vi "SVFA Unit Conversion (1 Ch).vi"(0 "spectrum":cluster{"x0":dbl, "dx":dbl, "magnitude":dbl[]} {"magnitude" format="%.2p"; "dx" format="%.2p"; "x0" format="%.2p"}, 1 "desired scaling":T2 {"dB reference (0: no change)" format="%.2f"}, 2 "spectral density desired":T1(ring), 4 "spectrum info in":T3={"channel name"="", "description"="", "x-axis units"=0, "spectral info"={"spectrum type"=enum."Power [Magnitude^2]", "linear/dB"=enum."linear", "window"=0, "window size"=0, "FFT size"=0}, "engineering units"=0, "custom label"="", "dB reference [EU]"=0.0, "peak units"=enum."rms", "weighting filter"=0, "spectral density?"=FALSE, "unit label"="", "spectrum skewed?"=FALSE, "complimentary spectrum units"=enum."none"} {"x-axis units" items=["Time (s)"=0, "Frequency-CB (Hz)"=1, "Frequency-CPB (Hz)"=1248, "Frequency-Arbitrary (Hz)"=2357, "Quefrency (s)"=2, "Revolutions (rev)"=3, "Order"=4, "Speed (RPM)"=11, "Speed (rad/s)"=21, "Index"=65535]; "weighting filter" items=["Linear", "A-weighting", "B-weighting", "C-weighting", "ITU-R 468-4", "Dolby", "CCITT", "C-message", "Wb", "Wc", "Wd", "We", "Wf", "Wh", "Wj", "Wk", "Wm", "AES17 20 kHz lowpass", "AES17 40 kHz lowpass", "AES17 20 kHz highpass", "AES17 40 kHz highpass"]; "dB reference [EU]" format="%.2f"; "engineering units" items=["custom..."=0, "V"=1, "A"=21, "C"=30, "pC"=31, "s"=32, "-"=29, "Pa"=2, "N"=20, "g"=3, "m/s^2"=4, "m/s"=5, "m"=6, "mm/s"=12, "mm"=13, "micron/s"=14, "micron"=15, "in/s^2"=7, "in/s"=8, "in"=9, "mil/s"=10, "mil"=11, "rad/s^2"=16, "rad/s"=17, "rad"=18, "deg/s^2"=26, "deg/s"=27, "deg"=28, "RPM"=22, "cycle/s^2"=23, "Hz"=24, "cycle"=25, "strain"=19]; "spectral info"."window" items=["None "=0, "Hanning"=1, "Hamming"=2, "Blackman-Harris"=3, "Exact Blackman"=4, "Blackman"=5, "Flat Top"=6, "4 Term B-Harris "=7, "7 Term B-Harris"=8, "Low Sidelobe"=9, "Force - Exponential"=10, "Gaussian"=62]}, 5 "error in (no error)":errorcluster) -> (14 "converted spectrum":cluster{"x0":dbl, "dx":dbl, "magnitude":dbl[]} {"magnitude" format="%.2p"; "dx" format="%.2p"; "x0" format="%.2p"}, 15 "unit label":string, 18 "spectrum info out":T3={"channel name"="", "description"="", "x-axis units"=0, "spectral info"={"spectrum type"=enum."Power [Magnitude^2]", "linear/dB"=enum."linear", "window"=0, "window size"=0, "FFT size"=0}, "engineering units"=0, "custom label"="", "dB reference [EU]"=0.0, "peak units"=enum."rms", "weighting filter"=0, "spectral density?"=FALSE, "unit label"="", "spectrum skewed?"=FALSE, "complimentary spectrum units"=enum."none"} {"x-axis units" items=["Time (s)"=0, "Frequency-CB (Hz)"=1, "Frequency-CPB (Hz)"=1248, "Frequency-Arbitrary (Hz)"=2357, "Quefrency (s)"=2, "Revolutions (rev)"=3, "Order"=4, "Speed (RPM)"=11, "Speed (rad/s)"=21, "Index"=65535]; "weighting filter" items=["Linear", "A-weighting", "B-weighting", "C-weighting", "ITU-R 468-4", "Dolby", "CCITT", "C-message", "Wb", "Wc", "Wd", "We", "Wf", "Wh", "Wj", "Wk", "Wm", "AES17 20 kHz lowpass", "AES17 40 kHz lowpass", "AES17 20 kHz highpass", "AES17 40 kHz highpass"]; "dB reference [EU]" format="%.2f"; "engineering units" items=["custom..."=0, "V"=1, "A"=21, "C"=30, "pC"=31, "s"=32, "-"=29, "Pa"=2, "N"=20, "g"=3, "m/s^2"=4, "m/s"=5, "m"=6, "mm/s"=12, "mm"=13, "micron/s"=14, "micron"=15, "in/s^2"=7, "in/s"=8, "in"=9, "mil/s"=10, "mil"=11, "rad/s^2"=16, "rad/s"=17, "rad"=18, "deg/s^2"=26, "deg/s"=27, "deg"=28, "RPM"=22, "cycle/s^2"=23, "Hz"=24, "cycle"=25, "strain"=19]; "spectral info"."window" items=["None "=0, "Hanning"=1, "Hamming"=2, "Blackman-Harris"=3, "Exact Blackman"=4, "Blackman"=5, "Flat Top"=6, "4 Term B-Harris "=7, "7 Term B-Harris"=8, "Low Sidelobe"=9, "Force - Exponential"=10, "Gaussian"=62]}, 19 "error out":errorcluster)   [LabVIEW 2017]
doc: "Converts between dB/linear, magnitude/magnitude^2, rms/peak/peak-peak, spectrum/spectral density, and dB ref1/dB ref2. Wire data to the <B>spectrum</B> input to determine the polymorphic instance to use or manually select the instance."
uses:
  <vilib>/addons/_NISVFA/_Shared subVIs/Controls/svc_Spectrum Info.ctl
  <vilib>/addons/_NISVFA/_Shared subVIs/Controls/svc_X-Axis Units.ctl
  <vilib>/addons/_NISVFA/_Shared subVIs/Controls/svc_Spectrum Type.ctl
  <vilib>/addons/_NISVFA/_Shared subVIs/Controls/svc_Engineering Units Text Ring.ctl
  <vilib>/addons/_NISVFA/_Shared subVIs/Controls/svc_Weighting Filter Text Ring.ctl
  <vilib>/addons/_NISVFA/_Shared subVIs/Controls/svc_Complimentary Spectrum Units.ctl
  <vilib>/addons/_NISVFA/_Spectrum Processing/subVIs/svfa_Peak to RMS to Peak2Peak.vi
  <vilib>/addons/_NISVFA/_Spectrum Processing/subVIs/svfa_Mag to Mag2.vi
  <vilib>/addons/_NISVFA/_Spectrum Processing/subVIs/svfa_Linear to dB.vi
  <vilib>/addons/_NISVFA/_Spectrum Processing/subVIs/svfa_dBrefA to dBrefB.vi
  <vilib>/addons/_NISVFA/_Spectrum Processing/subVIs/svfa_Spectrum to Spectral Density.vi
  <vilib>/addons/_NISVFA/_Shared subVIs/Common/svc_Get Weighting Enum and Labels.vi
  <vilib>/addons/_NISVFA/_Shared subVIs/Common/svc_Unit Label Lexical Class.vi
  <vilib>/addons/_NISVFA/_Shared subVIs/Common/svc_Engineering Units to Unit Label.vi
  <vilib>/addons/_NISVFA/_Shared subVIs/Common/svc_Format Value (DBL).vi
  <vilib>/addons/_NISVFA/_Shared subVIs/Common/svc_Window Parameters.vi
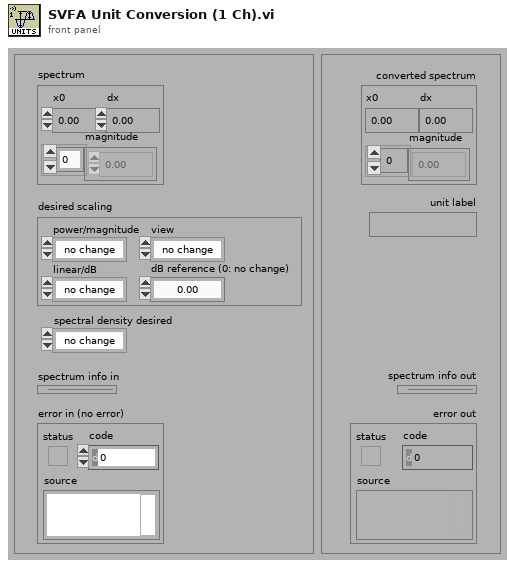
[diagram p1: front panel]
types:
  T1 = enum16{"no change", "spectrum", "spectral density"}
  T2 = cluster{"linear/dB":enum16{"no change", "linear", "dB"}, "dB reference (0: no change)":dbl, "power/magnitude":enum16{"no change", "power", "magnitude"}, "view":enum16{"no change", "rms", "peak", "peak-peak"}}
  T3 = typedef "svc_Spectrum Info.ctl" = cluster{"channel name":string, "description":string, "x-axis units":T4, "spectral info":cluster{"spectrum type":T5, "linear/dB":enum16{"linear", "dB"}, "window":u16, "window size":i32, "FFT size":i32}, "engineering units":T6, "custom label":string, "dB reference [EU]":dbl, "peak units":enum16{"rms", "peak", "peak-peak"}, "weighting filter":T7, "spectral density?":bool, "unit label":string, "spectrum skewed?":bool, "complimentary spectrum units":T8}
  T4 = typedef "svc_X-Axis Units.ctl" = u16
  T5 = typedef "svc_Spectrum Type.ctl" = enum16{"FFT Spectrum [complex]", "Amplitude [Magnitude]", "Power [Magnitude^2]", "Cross Spectrum [complex]", "Frequency Response [Complex]"}
  T6 = typedef "svc_Engineering Units Text Ring.ctl" = u16
  T7 = typedef "svc_Weighting Filter Text Ring.ctl" = u16
  T8 = typedef "svc_Complimentary Spectrum Units.ctl" = enum16{"none", "radians", "degrees", "cycles", "imaginary"}
  T9 = cluster{"linear/dB":bool, "dB reference (0: no change)":bool, "power/magnitude":bool, "view":bool}
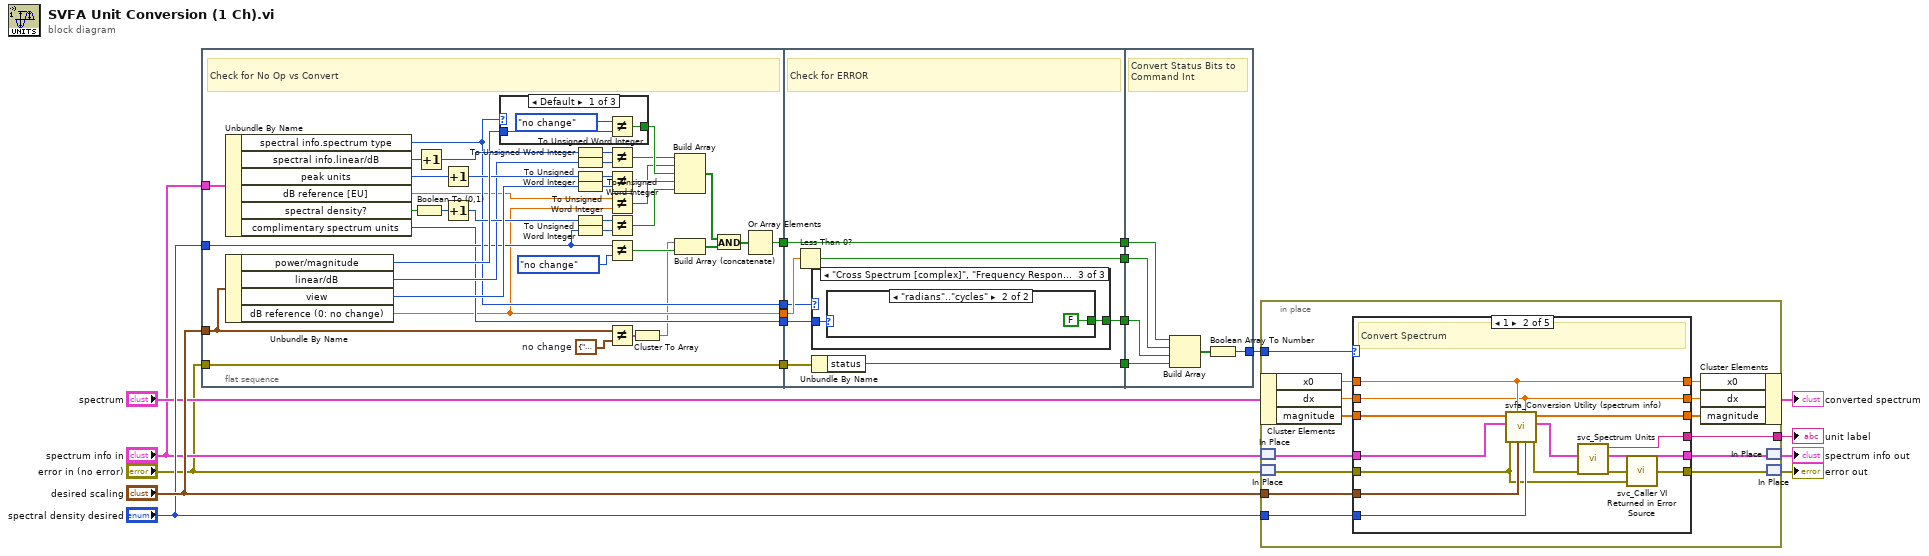
[diagram p0: block diagram]
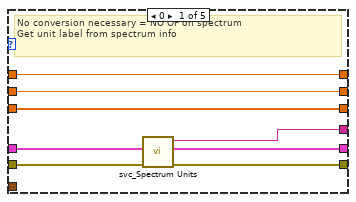
[diagram p2: hidden frame]
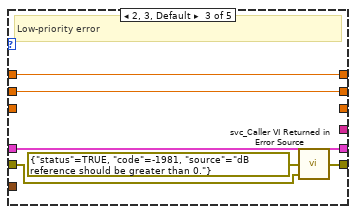
[diagram p3: hidden frame]
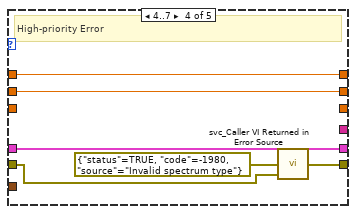
[diagram p4: hidden frame]
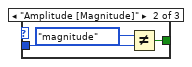
[diagram p6: hidden frame]
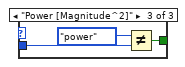
[diagram p7: hidden frame]
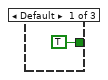
[diagram p8: hidden frame]
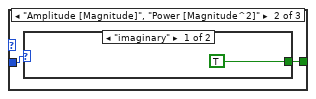
[diagram p9: hidden frame]
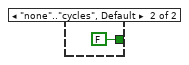
[diagram p10: hidden frame]
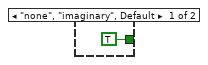
[diagram p11: hidden frame]
diagram:
  n1 = flat-sequence "Check for No Op vs Convert" {
    tunnel: "desired scaling" -> [w39]
    tunnel: "spectrum info in" -> [w57]
    tunnel: "spectral density desired" -> [w36]
    tunnel: [w30] -> w14
    tunnel: [w32] -> w13
    tunnel: [w34] -> w12
    tunnel: [w37] -> w11
    tunnel: "error in (no error)" -> [w35]
    tunnel: [w35] -> w1
    tunnel: w14 -> [w74]
    tunnel: w13 -> [w73]
    tunnel: w12 -> [w72]
    tunnel: w11 -> [w71]
    tunnel: [w74] -> w7
    tunnel: [w70] -> w6
    tunnel: [w69] -> w5
    tunnel: [w68] -> w4
    tunnel: w1 -> [w67]
    tunnel: w7 -> [w85]
    tunnel: w6 -> [w86]
    tunnel: w5 -> [w87]
    tunnel: w4 -> [w88]
    tunnel: [w84] -> w3
    frame #0 {
      w56 = T2 {"linear/dB"=enum."no change", "dB reference (0: no change)"=0.0, "power/magnitude"=enum."no change", "view"=enum."no change"}  # no change
      # "Check for No Op vs Convert"
      n2 = Unbundle By Name(w57) -> ("spectral info.spectrum type"=w37:T5, "spectral info.linear/dB"=w54:enum16{"linear", "dB"}, "peak units"=w47:enum16{"rms", "peak", "peak-peak"}, "dB reference [EU]"=w33:dbl, "spectral density?"=w46:bool, "complimentary spectrum units"=w34:T8)
      n3 = Unbundle By Name(w39) -> ("power/magnitude"=w51:enum16{"no change", "power", "magnitude"}, "linear/dB"=w38:enum16{"no change", "linear", "dB"}, "view"=w49:enum16{"no change", "rms", "peak", "peak-peak"}, "dB reference (0: no change)"=w32:dbl)
      n4 = Boolean To (0,1)(Boolean=w46) -> (0, 1=w44:i16)
      n5 = Increment(x=w54) -> (x+1=w53:enum16{"linear", "dB"})
      n6 = Increment(x=w47) -> (x+1=w48:enum16{"rms", "peak", "peak-peak"})
      n7 = Increment(x=w44) -> (x+1=w43:i16)
      n8 = case shown="Default" w37 {
        tunnel: [w58 w61 w64] -> w27
        tunnel: w51 -> [w60 w63 w66]
        frame Default {
          n9 = Not Equal?(x=enum16{"no change", "power", "magnitude"}."no change", y=w60) -> (x != y?=w58:bool)
        }
        frame "Amplitude [Magnitude]" {
          n10 = Not Equal?(x=enum16{"no change", "power", "magnitude"}."magnitude", y=w63) -> (x != y?=w61:bool)
        }
        frame "Power [Magnitude^2]" {
          n11 = Not Equal?(x=enum16{"no change", "power", "magnitude"}."power", y=w66) -> (x != y?=w64:bool)
        }
      }
      n12 = To Unsigned Word Integer(number=w53) -> (unsigned 16bit integer=w50:u16)
      n13 = To Unsigned Word Integer(number=w38) -> (unsigned 16bit integer=w52:u16)
      n14 = To Unsigned Word Integer(number=w48) -> (unsigned 16bit integer=w45:u16)
      n15 = To Unsigned Word Integer(number=w49) -> (unsigned 16bit integer=w41:u16)
      n16 = To Unsigned Word Integer(number=w43) -> (unsigned 16bit integer=w42:u16)
      n17 = To Unsigned Word Integer(number=w36) -> (unsigned 16bit integer=w40:u16)
      n18 = Not Equal?(x=w50, y=w52) -> (x != y?=w21:bool)
      n19 = Not Equal?(x=w45, y=w41) -> (x != y?=w26:bool)
      n20 = Not Equal?(x=w33, y=w32) -> (x != y?=w20:bool)
      n21 = Not Equal?(x=w42, y=w40) -> (x != y?=w25:bool)
      n22 = Not Equal?(x=w36, y=T1."no change" ("spectral density desired")) -> (x != y?=w29:bool)
      n23 = Not Equal?(x=w39, y=w56) -> (x != y?=w31:T9)
      n24 = Cluster To Array(cluster=w31) -> (array=w28:bool[])
      n25 = Build Array(w21, w20, w27, w26, w25) -> (w23:bool[])
      n26 = Build Array (concatenate)(w28, w29) -> (w24:bool[])
      n27 = And(x=w23, y=w24) -> (x .and. y?=w22:bool[])
      n28 = Or Array Elements(Boolean array=w22) -> (logical OR=w30:bool)
    }
    frame #1 {
      # "Check for ERROR"
      n29 = Less Than 0?(x=w73) -> (x < 0?=w70:bool)
      n30 = case shown="\"Cross Spectrum [complex]\", \"Frequency Response [Complex]\"" w71 {
        tunnel: [TRUE ("status") w76 w80] -> w69
        tunnel: w72 -> [_ w77 w81]
        frame Default {
        }
        frame "Amplitude [Magnitude]", "Power [Magnitude^2]" {
          n31 = case shown="\"imaginary\"" w77 {
            tunnel: [TRUE ("status") FALSE ("status")] -> w76
            frame "imaginary" {
            }
            frame "none".."cycles", Default {
            }
          }
        }
        frame "Cross Spectrum [complex]", "Frequency Response [Complex]" {
          n32 = case shown="\"radians\"..\"cycles\"" w81 {
            tunnel: [TRUE ("status") FALSE ("status")] -> w80
            frame "none", "imaginary", Default {
            }
            frame "radians".."cycles" {
            }
          }
        }
      }
      n33 = Unbundle By Name(w67) -> ("status"=w68:bool)
    }
    frame #2 {
      # "Convert Status Bits to Command Int"
      n34 = Build Array(w85, w86, w87, w88) -> (w89:bool[])
      n35 = Boolean Array To Number(Boolean array=w89) -> (number=w84:u32)
    }
  }
  n36 = in-place {
    in-place-border: "desired scaling" -> [w103]
    in-place-border: [w102] -> w18
    in-place-border: "spectral density desired" -> [w101]
    in-place-border: w3 -> [w100]
    n37 = in-place-cluster #1("spectrum") -> ("x0"=w99:dbl, "dx"=w98:dbl, "magnitude"=w97:dbl[])
    n38 = in-place-match #2("spectrum info in") -> (w93:T3)
    n39 = in-place-match #3("error in (no error)") -> (w90:errorcluster)
    n40 = case shown="1" w100 {
      tunnel: w90 -> [w108 w116 w128 w136 w141]
      tunnel: w103 -> [_ w125 _ _ _]
      tunnel: [w107 w118 w129 w135 w141] -> w91
      tunnel: [w109 w124 _ _ _] -> w102
      tunnel: [w110 w123 w131 w134 w140] -> w92
      tunnel: w93 -> [w111 w122 w131 w134 w140]
      tunnel: w101 -> [_ w121 _ _ _]
      tunnel: [w106 w113 w127 w132 w139] -> w96
      tunnel: w99 -> [w106 w113 w127 w132 w139]
      tunnel: [w105 w112 w126 w133 w138] -> w95
      tunnel: w98 -> [w105 w112 w126 w133 w138]
      tunnel: [w104 w114 _ _ _] -> w94
      tunnel: w97 -> [w104 w115 _ _ _]
      frame 0 {
        # "No conversion necessary = NO OP on spectrum\nGet unit label from spectrum info"
        n41 = call <vilib>:"svc_Spectrum Units.vi"("error in (no error)"=w108, "spectrum info in"=w111) -> ("error out"=w107:errorcluster, "spectrum info out"=w110:T3, "unit label"=w109:string)  [unwired: 2 in, 1 out]
      }
      frame 1 {
        # "Convert Spectrum"
        n42 = call <vilib>:"svfa_Conversion Utility (spectrum info).vi"("spectral density desired"=w121, "dx"=w112, "desired scaling"=w125, "x0"=w113, "error in (no error)"=w116, "spectrum info in"=w122, "input signal"=w115) -> ("error out"=w120:errorcluster, "spectrum info out"=w119:T3, "converted signal"=w114:dbl[])  [unwired: 2 in]
        n43 = call <vilib>:"svc_Spectrum Units.vi"("error in (no error)"=w120, "spectrum info in"=w119) -> ("error out"=w117:errorcluster, "spectrum info out"=w123:T3, "unit label"=w124:string)  [unwired: 2 in, 1 out]
        n44 = call <vilib>:"svc_Caller VI Returned in Error Source.vi"("warning input to caller"=w116, "error in (no error)"=w117) -> ("error out"=w118:errorcluster)  [unwired: 3 in]
      }
      frame 2, 3, Default {
        # "Low-priority error"
        n45 = call <vilib>:"svc_Caller VI Returned in Error Source.vi"("warning input to caller"=w128, "error in (no error)"=errorcluster {"status"=TRUE, "code"=-1981, "source"="dB reference should be greater than 0."} ("error out")) -> ("error out"=w129:errorcluster)  [unwired: 3 in]
      }
      frame 4..7 {
        # "High-priority Error"
        n46 = call <vilib>:"svc_Caller VI Returned in Error Source.vi"("warning input to caller"=w136, "error in (no error)"=errorcluster {"status"=TRUE, "code"=-1980, "source"="Invalid spectrum type"} ("error out")) -> ("error out"=w135:errorcluster)  [unwired: 3 in]
      }
      frame 8..15 {
        # "Input error"
      }
    }
    n47 = in-place-cluster #1("x0"=w96, "dx"=w95, "magnitude"=w94) -> (→"converted spectrum":cluster{"x0":dbl, "dx":dbl, "magnitude":dbl[]})
    n48 = in-place-match #2(w92) -> (→"spectrum info out":T3)
    n49 = in-place-match #3(w91) -> (→"error out":errorcluster)
  }
  "unit label" <- w18
